vi "Trige.vi"() -> ()   [LabVIEW 2017]
panel:
  out "Trigle_3":bool
  out "Trigle_2":bool
  out "Trigle_1":bool
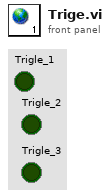
[diagram p1: front panel]
diagram:
